vi "Execute.vi"(8 "error in":errorcluster, 11 "Filter Step in":refnum<class "Filter Step.lvclass">) -> (0 "error out":errorcluster, 1 "Next Step?":bool, 2 "MSG":string, 3 "Filter Step out":refnum<class "Filter Step.lvclass">)   [LabVIEW 2016, in "Controller.lvlib" / "Filter Step.lvclass"]
uses:
  Filter Step.lvclass
  Filter Step.lvclass/Filter Step.ctl
  Messages/Change Filter MSG/Change Filter Position MSG.lvclass
  C:/Program Files (x86)/National Instruments/LabVIEW 2016/vi.lib/ActorFramework/Message/Message.lvclass
  Messages/Change Filter MSG/Change Filter Position MSG.lvclass/Change Filter Position MSG.ctl
  <vilib>/ActorFramework/Message Enqueuer/Message Enqueuer.lvclass/Message Enqueuer.ctl
  Messages/Change Filter MSG/Write Cell.vi
  <vilib>/ActorFramework/Message Priority Queue/Priority Enqueue.vi
  gController.lvclass
  <vilib>/ActorFramework/Message Enqueuer/Message Enqueuer.lvclass
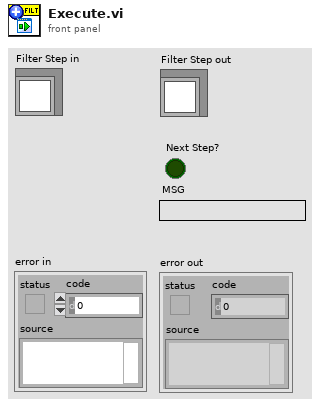
[diagram p1: front panel]
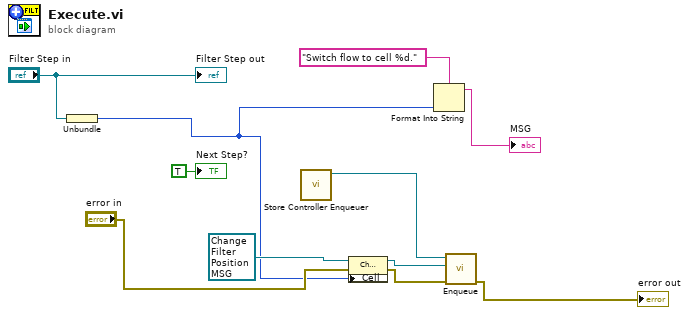
[diagram p0: block diagram]
diagram:
  n1 = Unbundle("Filter Step in") -> (w2:u8)
  n2 = call "Store Controller Enqueuer.vi"() -> ("Controller Enqueuer Out"=w7:refnum<class "Message Enqueuer.lvclass">)  [unwired: 11 in]
  n3 = property class="Change Filter Position"(reference=refnum<class "Change Filter Position MSG.lvclass"> refnum ("Controller.lvlib:Change Filter Position"), error in="error in", "Cell"=w2) -> (reference out=w6:refnum<class "Change Filter Position MSG.lvclass">, error out=w5:errorcluster)
  n4 = Format Into String(format string="Switch flow to cell %d.", w2) -> (resulting string=→"MSG":string)  [unwired: 2 in, 1 out]
  n5 = call <vilib>:"Enqueue.vi"("error in (no error)"=w5, "Message"=w6, "Message Enqueuer in"=w7) -> ("error out"=→"error out":errorcluster)  [unwired: 7 in, 1 out]
  "Filter Step out" <- "Filter Step in"
  "Next Step?" <- TRUE ("Next Step?")
